vi "Define_Column_Number_101_Case-1.vi"(1 "[IN] Current index":i32, 2 "[IN] Index of \nSubtrack Row":i32) -> (0 "[OUT] Column for subtrack":i32)   [LabVIEW 2013]
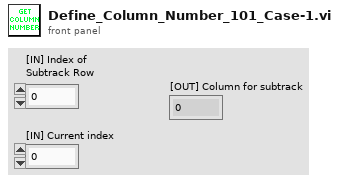
[diagram p1: front panel]
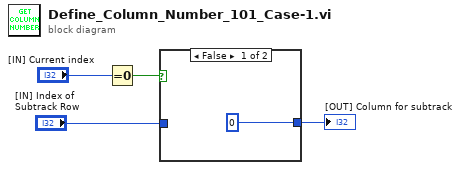
[diagram p0: block diagram]
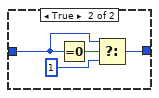
[diagram p2: hidden frame]
diagram:
  n1 = Equal To 0?(x="[IN] Current index") -> (x = 0?=w3:bool)
  n2 = case shown="False" w3 {
    tunnel: "[IN] Index of \nSubtrack Row" -> [_ w7]
    tunnel: [0 ("f") w6] -> w1
    frame False {
    }
    frame True {
      n3 = Equal To 0?(x=w7) -> (x = 0?=w9:bool)
      n4 = Select(t=w7, s=w9, f=1) -> (s? t:f=w6:i32)
    }
  }
  "[OUT] Column for subtrack" <- w1
